vi "251213_Nikon_CheckStatus_XY stage.vi"(8 "error in":errorcluster caption="entrée d'erreur", 11 "NikonTi2AxLib.INikonTi2AxMicroscope":refnum<k7>) -> (0 "error out":errorcluster={"status"=TRUE, "code"=-9, "source"="Exception occured in Nikon.Ti2.Microscope.1: Failed in 231026_NikonTi2_Indicators_v2.vi"} caption="sortie d'erreur", 2 "XY stage cluster":T1, 3 "reference out":refnum<k7>)   [LabVIEW 2025]
doc: "This vi checks the current status of the microscope. One can add some extra devices such as fluorescence cube turret.\nThe automation should be open and close outside of this vi"
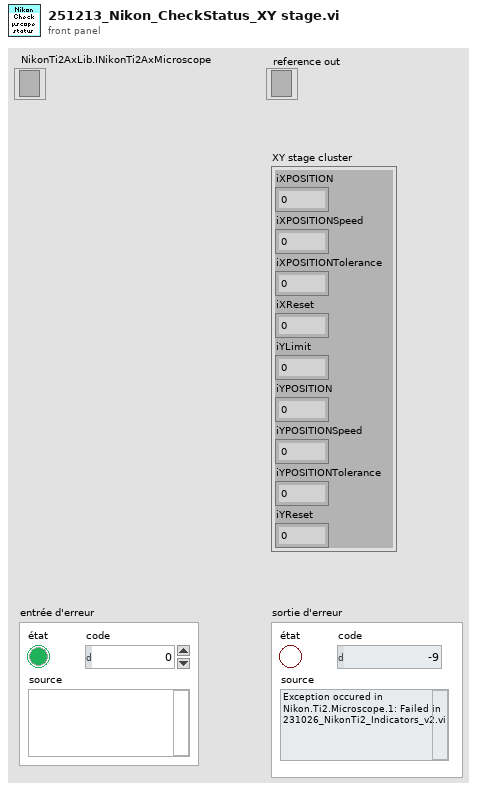
[diagram p1: front panel]
types:
  T1 = cluster{"iXPOSITION":i32, "iXPOSITIONSpeed":i32, "iXPOSITIONTolerance":i32, "iXReset":i32, "iYLimit":i32, "iYPOSITION":i32, "iYPOSITIONSpeed":i32, "iYPOSITIONTolerance":i32, "iYReset":i32}
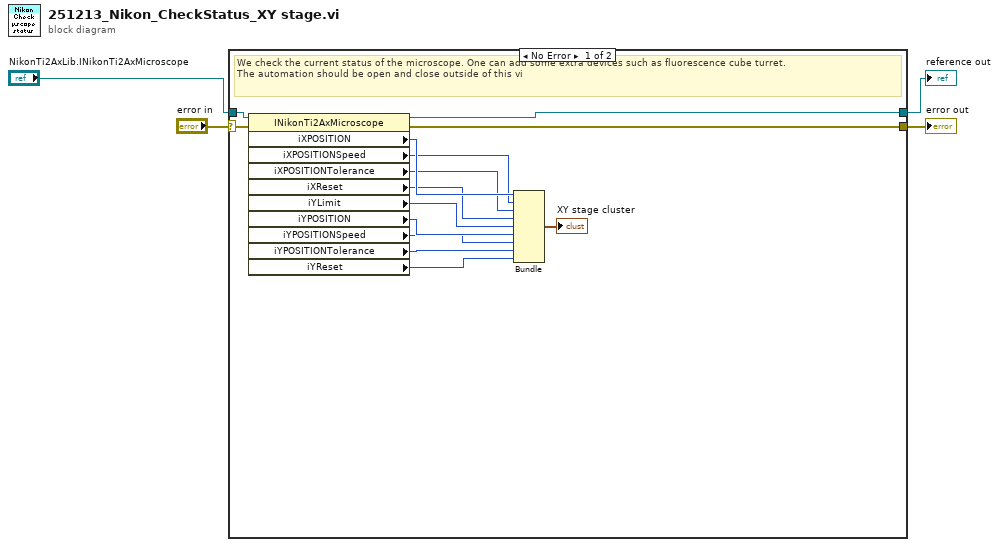
[diagram p0: block diagram]
diagram:
  n1 = case shown="No Error" "error in" {
    selector: "error in" -> [w17 w20]
    tunnel: [w16 w20] -> w3
    tunnel: "NikonTi2AxLib.INikonTi2AxMicroscope" -> [w18 w19]
    tunnel: [w15 w19] -> w2
    frame No Error {
      # "We check the current status of the microscope. One can add some extra devices such as fluorescence cube turret.\nThe automation should be open and close outside of this vi"
      n2 = property class="INikonTi2AxMicroscope"(reference=w18, error in=w17) -> (reference out=w15:refnum<k7>, error out=w16:errorcluster, "iXPOSITION"=w14:i32, "iXPOSITIONSpeed"=w13:i32, "iXPOSITIONTolerance"=w12:i32, "iXReset"=w11:i32, "iYLimit"=w10:i32, "iYPOSITION"=w9:i32, "iYPOSITIONSpeed"=w8:i32, "iYPOSITIONTolerance"=w7:i32, "iYReset"=w6:i32)
      n3 = Bundle("iXPOSITION"=w14, "iXPOSITIONSpeed"=w13, "iXPOSITIONTolerance"=w12, "iXReset"=w11, "iYLimit"=w10, "iYPOSITION"=w9, "iYPOSITIONSpeed"=w8, "iYPOSITIONTolerance"=w7, "iYReset"=w6) -> (→"XY stage cluster":T1)  [unwired: 1 in]
    }
    frame Error {
    }
  }
  "error out" <- w3
  "reference out" <- w2
